vi "I-SRC Test Communications (26XX).vi"(8 "error in (no error)":errorcluster, 11 "VISA resource name in":refnum<visa-resource-name>) -> (0 "error out":errorcluster, 3 "VISA resource name out":refnum<visa-resource-name>)   [LabVIEW 2016, in "Hall Effect Library.lvlib"]
uses:
  Hall Effect Library.lvlib
  <instrlib>/KE26XX/KE26XX.lvlib
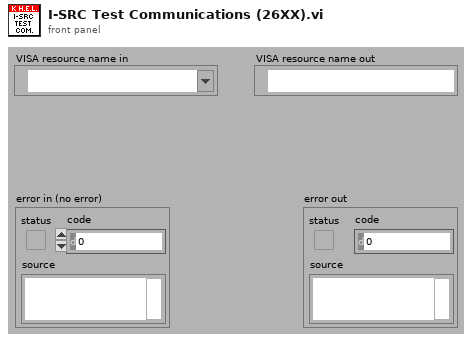
[diagram p1: front panel]
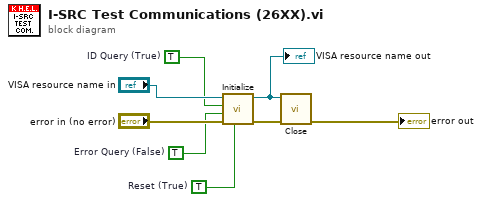
[diagram p0: block diagram]
diagram:
  w2 = TRUE  # Reset (True)
  w3 = TRUE  # Error Query (False)
  w4 = TRUE  # ID Query (True)
  n1 = call <instrlib>:"Initialize.vi"("Reset (True)"=w2, "error in (no error)"="error in (no error)", "Error Query (False)"=w3, "ID Query (True)"=w4, "VISA resource name"="VISA resource name in") -> ("error out"=w8:errorcluster, "VISA resource name out"=w1:refnum<visa-resource-name>)  [unwired: 1 in, 4 out]
  "VISA resource name out" <- w1
  n2 = call <instrlib>:"Close.vi"("error in (no error)"=w8, "VISA resource name"=w1) -> ("error out"=→"error out":errorcluster)  [unwired: 9 out]
